vi "Pre Launch Init.vi"(11 "VIStore in":refnum<class "VIStore.lvclass">) -> (0 "error out":errorcluster, 3 "VIStore out":refnum<class "VIStore.lvclass">)   [LabVIEW 2015, in "VI App Store.lvlib" / "VIStore.lvclass"]
doc: "(<B>Filename</B>: Actor Framework.lvlib:Actor.lvclass:Pre Launch Init.vi)\n\nDefines behavior that occurs after the Launch Nested Actor method is invoked but before the actor's Actor Core method begins running.\n\nBy default, this method does nothing. A descendant class may override it to define behavior."
uses:
  VIStore.lvclass
  VIStore.lvclass/VIStore.ctl
  <vilib>/Utility/config.llb/NI_LVConfig.lvlib
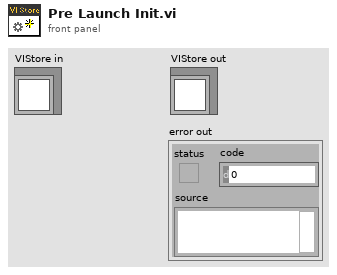
[diagram p1: front panel]
types:
  T1 = typedef "Item Actor.lvlib/Settings.lvclass/Settings Data.ctl" = cluster{"Categories Path":path, "Resizable":bool}
  T2 = typedef "NI_LVConfig.lvlib/Config Data RefNum.ctl" = refnum<k1>
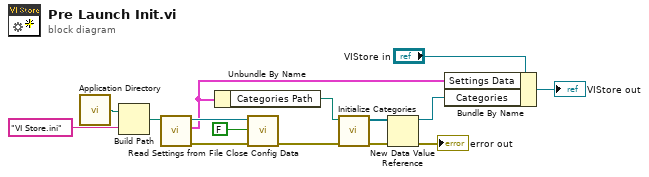
[diagram p0: block diagram]
diagram:
  n1 = call <vilib>:"Application Directory.vi"() -> ("Application Directory"=w15:path)
  n2 = Build Path(base path=w15, name or relative path="VI Store.ini") -> (appended path=w13:path)
  n3 = call "Read Settings from File.vi"("Ini path"=w13) -> ("error out"=w8:errorcluster, "Store Settings"=w2:T1, "Ini out"=w12:T2)  [unwired: 8 in]
  n4 = Unbundle By Name(w2) -> ("Categories Path"=w1:path)
  n5 = call <vilib>:"Close Config Data.vi"("error in (no error)"=w8, "write file if changed (T)"=FALSE, "refnum"=w12) -> ("error out"=w7:errorcluster)  [unwired: 7 in, 1 out]
  n6 = call "Initialize Categories.vi"("error in (no error)"=w7, "Cats XML"=w1) -> ("error out"=w4:errorcluster, "All Categories"=w6:refnum<class "Category.lvclass">[])  [unwired: 8 in]
  n7 = New Data Value Reference(data value=w6, error in=w4) -> (data value reference=w5:refnum<data-value>, error out=→"error out":errorcluster)
  n8 = Bundle By Name(cluster="VIStore in", "Settings Data"=w2, "Categories"=w5) -> (→"VIStore out":refnum<class "VIStore.lvclass">)
